vi "Parse List Objects Result.vi"(8 "error in (no error)":errorcluster, 10 "Response body":string) -> (0 "error out":errorcluster, 3 "List Objects Result":T1)   [LabVIEW 2015, in "NI_AWS_S3.lvlib" / "Object.lvlib"]
doc: "Parse out the Results from the Response body of a List bucket request."
uses:
  Object.lvlib
  List Objects Result.ctl
  Object Content.ctl
  Storage Class.ctl
  Owner.ctl
  Common Prefix.ctl
  NI_AWS_S3.lvlib
  XML Parsing/NI_XML Parsing.lvlib
  Core/NI_AWS_Core.lvlib
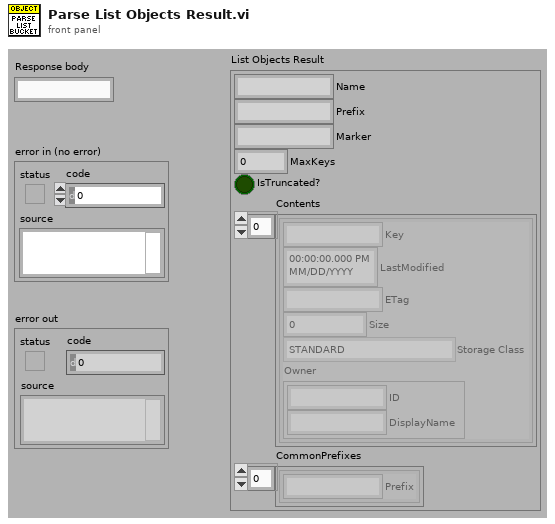
[diagram p1: front panel]
types:
  T1 = typedef "NI_AWS_S3.lvlib/List Objects Result.ctl" = cluster{"Name":string, "Prefix":string, "Marker":string, "MaxKeys":u16, "IsTruncated?":bool, "Contents":T2[], "CommonPrefixes":T5[]}
  T2 = typedef "NI_AWS_S3.lvlib/Object Content.ctl" = cluster{"Key":string, "LastModified":timestamp, "ETag":string, "Size":u64, "Storage Class":T3, "Owner":T4}
  T3 = typedef "NI_AWS_S3.lvlib/Storage Class.ctl" = enum16{"STANDARD", "REDUCED_REDUNDANCY"}
  T4 = typedef "NI_AWS_S3.lvlib/Owner.ctl" = cluster{"ID":string, "DisplayName":string}
  T5 = typedef "NI_AWS_S3.lvlib/Common Prefix.ctl" = cluster{"Prefix":string}
  T6 = cluster{"[0]":string, "[1]":string, "[2]":string, "[3]":string, "[4]":string}
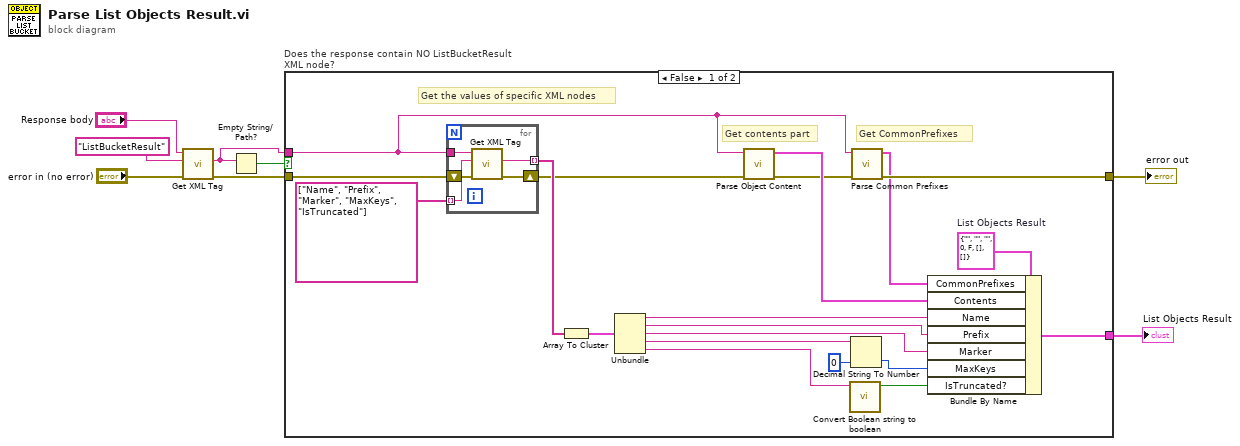
[diagram p0: block diagram]
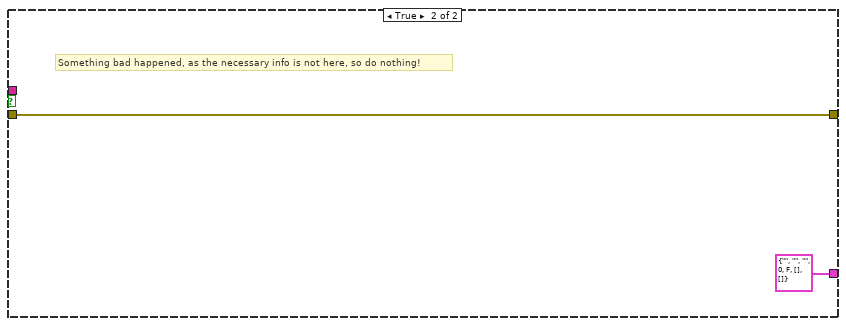
[diagram p2: hidden frame]
diagram:
  n1 = call "Get XML Tag.vi"("error in (no error)"="error in (no error)", "Tag name"="ListBucketResult", "XML String in"="Response body") -> ("error out"=w2:errorcluster, "Tag value"=w1:string)  [unwired: 4 in, 3 out]
  n2 = Empty String/Path?(string/path=w1) -> (empty?=w3:bool)
  n3 = case "Does the response contain NO ListBucketResult XML node?" shown="False" w3 {
    tunnel: w1 -> [w9 _]
    tunnel: w2 -> [w20 w35]
    tunnel: [w27 T1 {"Name"="", "Prefix"="", "Marker"="", "MaxKeys"=0, "IsTruncated?"=FALSE, "Contents"=[], "CommonPrefixes"=[]} ("ListBucketResult")] -> w8
    tunnel: [w24 w35] -> w7
    frame False {
      w22 = T1 {"Name"="", "Prefix"="", "Marker"="", "MaxKeys"=0, "IsTruncated?"=FALSE, "Contents"=[], "CommonPrefixes"=[]}  # List Objects Result
      # "Get the values of specific XML nodes"
      # "Get CommonPrefixes"
      # "Get contents part"
      n4 = for {
        tunnel: string[] ["Name", "Prefix", "Marker", "MaxKeys", "IsTruncated"] -> [w32] mode=indexing
        tunnel: w9 -> [w31]
        tunnel: [w30] -> w19 mode=indexing
        shift-right: [w29] -> w10
        shift-left: w20 -> [w33]
        n5 = call "Get XML Tag.vi"("error in (no error)"=w33, "Tag name"=w32, "XML String in"=w31) -> ("error out"=w29:errorcluster, "Tag value"=w30:string)  [unwired: 4 in, 3 out]
      }
      n6 = Array To Cluster(array=w19) -> (cluster=w18:T6)
      n7 = Unbundle(w18) -> ("[0]"=w17:string, "[1]"=w16:string, "[2]"=w15:string, "[3]"=w14:string, "[4]"=w12:string)
      n8 = call "Parse Object Content.vi"("error in (no error)"=w10, "Response body"=w9) -> ("error out"=w25:errorcluster, "Object content"=w26:T2[])  [unwired: 8 in]
      n9 = call "Convert Boolean string to boolean.vi"("Boolean String"=w12) -> ("Boolean"=w11:bool)  [unwired: 10 in]
      n10 = Decimal String To Number(string=w14, default (0L)=u16 0) -> (number=w13:u16)  [unwired: 1 in, 1 out]
      n11 = call "Parse Common Prefixes.vi"("error in (no error)"=w25, "Response body"=w9) -> ("error out"=w24:errorcluster, "Common Prefixes"=w23:T5[])  [unwired: 8 in]
      n12 = Bundle By Name(cluster=w22, "CommonPrefixes"=w23, "Contents"=w26, "Name"=w17, "Prefix"=w16, "Marker"=w15, "MaxKeys"=w13, "IsTruncated?"=w11) -> (w27:T1)
    }
    frame True {
      # "Something bad happened, as the necessary info is not here, so do nothing!"
    }
  }
  "List Objects Result" <- w8
  "error out" <- w7
